vi "Notifier_Operation_Select.vi"() -> ()   [LabVIEW 2023]
uses:
  Control 1.ctl
panel:
  out "Latest_Notification":bool
  in  "Notifier_Name":string
  out "Error_Out":errorcluster
  in  "Error_In":errorcluster
  in  "Notifier_Operation_Select":T1=enum."Release_Notifier"
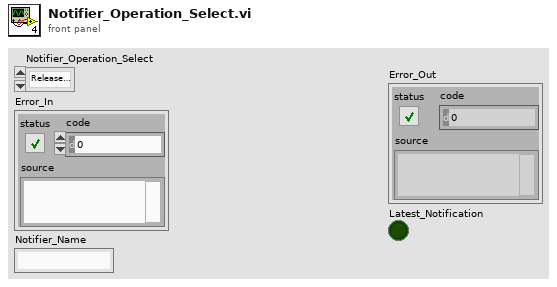
[diagram p1: front panel]
types:
  T1 = typedef "Control 1.ctl" = enum16{"Obtain_Notifier", "Send_Notification", "Get_Notification_Status", "Release_Notifier"}
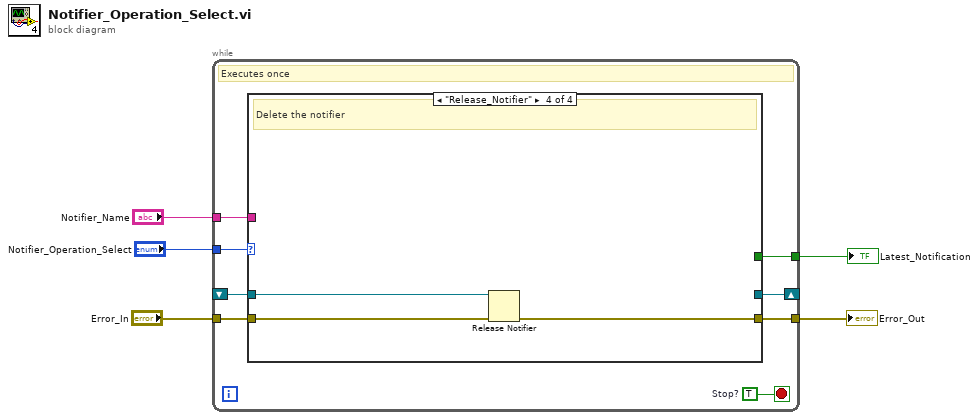
[diagram p0: block diagram]
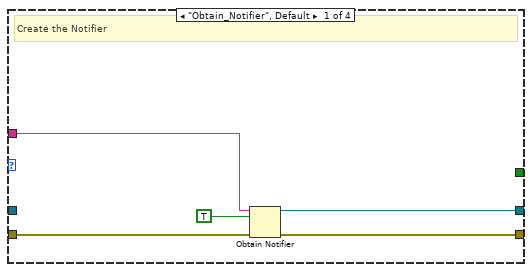
[diagram p2: hidden frame]
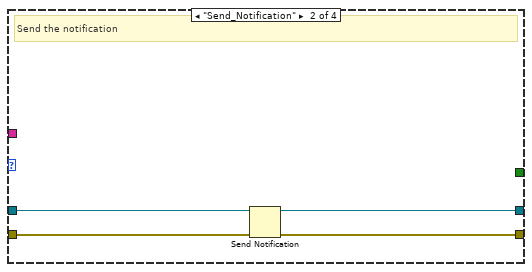
[diagram p3: hidden frame]
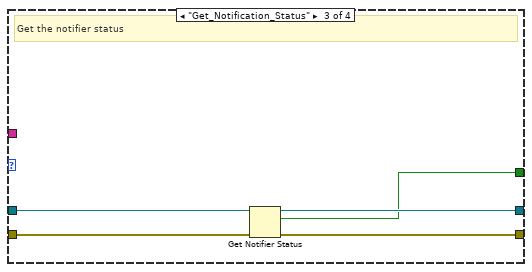
[diagram p4: hidden frame]
diagram:
  n1 = while {
    tunnel: "Notifier_Operation_Select" -> [w13]
    tunnel: "Error_In" -> [w12]
    tunnel: [w11] -> w3
    shift-right: [w10] -> _
    shift-left: _ -> [w9]
    tunnel: "Notifier_Name" -> [w8]
    tunnel: [w7] -> w1
    stop <- w6 stop-if-true
    w6 = TRUE  # Stop?
    # "Executes once"
    n2 = case shown="\"Release_Notifier\"" w13 {
      tunnel: w12 -> [w18 w22 w27 w30]
      tunnel: [w17 w21 w26 w29] -> w11
      tunnel: [w14 w20 w24 _] -> w10
      tunnel: w9 -> [_ w19 w25 w28]
      tunnel: w8 -> [w16 _ _ _]
      tunnel: [_ _ w23 _] -> w7
      frame "Obtain_Notifier", Default {
        # "Create the Notifier"
        n3 = Obtain Notifier(name (unnamed)=w16, notification data type=TRUE, error in (no error)=w18) -> (notifier out=w14:refnum<notifier>, error out=w17:errorcluster)  [unwired: 1 in, 1 out]
      }
      frame "Send_Notification" {
        # "Send the notification"
        n4 = Send Notification(notifier=w19, error in (no error)=w22) -> (notifier out=w20:refnum<notifier>, error out=w21:errorcluster)  [unwired: 1 in]
      }
      frame "Get_Notification_Status" {
        # "Get the notifier status"
        n5 = Get Notifier Status(notifier=w25, error in (no error)=w27) -> (notifier out=w24:refnum<notifier>, current notification=w23:bool, error out=w26:errorcluster)  [unwired: 2 out]
      }
      frame "Release_Notifier" {
        # "Delete the notifier"
        n6 = Release Notifier(notifier=w28, error in (no error)=w30) -> (error out=w29:errorcluster)  [unwired: 1 in, 2 out]
      }
    }
  }
  "Error_Out" <- w3
  "Latest_Notification" <- w1
